vi "_f_SerialComm_Hardware_Module.vi"(5 "Enable(T)":bool=TRUE, 7 "Command":T1, 8 "error in (no error)":errorcluster, 9 "Bytes to read":u32, 10 "Write string":string, 11 "VISA resource name":refnum<visa-resource-name>) -> (0 "error out":errorcluster, 1 "Bytes?":u32, 2 "Read string":string)   [LabVIEW 2013]
uses:
  _f_SerialComm_Hardware_Module Control.ctl
  <vilib>/Instr/_visa.llb/VISA Configure Serial Port (Instr).vi
panel:
  # "Input Data"
  # "Output Data"
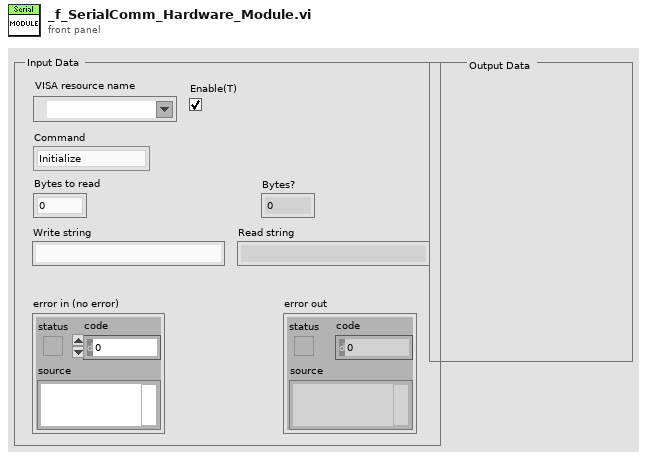
[diagram p1: front panel]
types:
  T1 = typedef "_f_SerialComm_Hardware_Module Control.ctl" = enum16{"Initialize", "Write", "Bytes?", "Read", "Shutdown"}
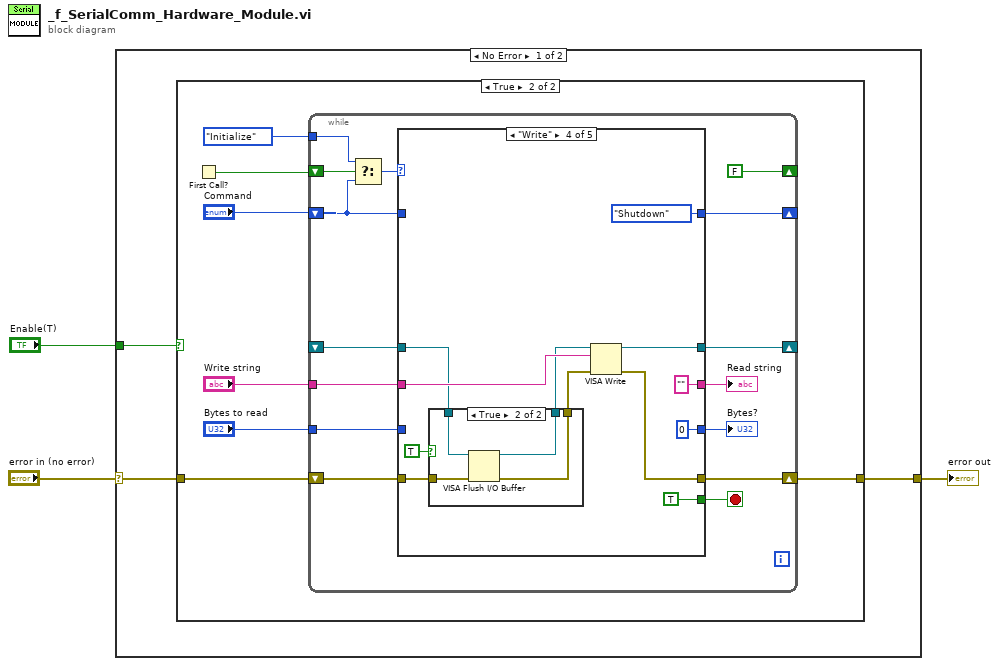
[diagram p0: block diagram]
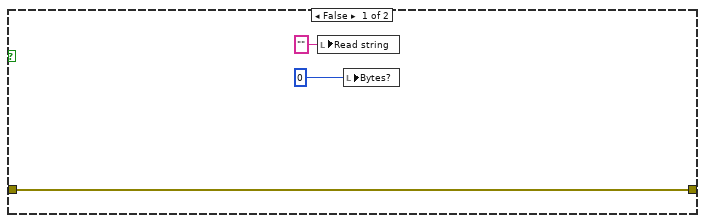
[diagram p2: hidden frame]
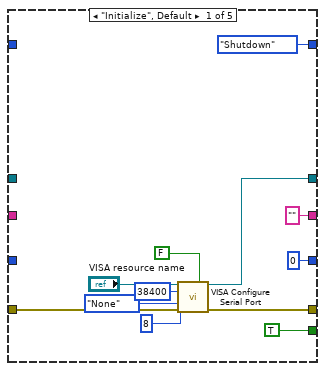
[diagram p3: hidden frame]
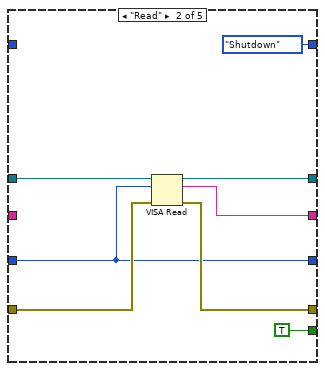
[diagram p4: hidden frame]
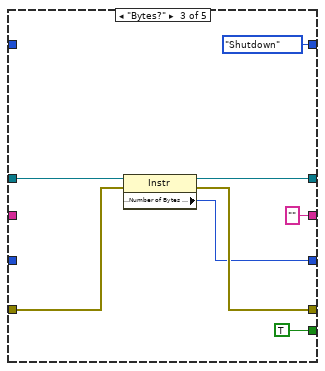
[diagram p5: hidden frame]
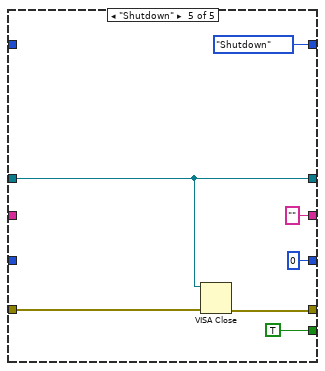
[diagram p7: hidden frame]
diagram:
  n1 = case shown="No Error" "error in (no error)" {
    selector: "error in (no error)" -> [w6 w85]
    tunnel: [w5 w85] -> w2
    tunnel: "Enable(T)" -> [w4 _]
    frame No Error {
      n2 = case shown="True" w4 {
        tunnel: w6 -> [w9 w14]
        tunnel: [w9 w13] -> w5
        frame False {
          n3 = local write "Read string"("" ("Read string")) -> ()
          n4 = local write "Bytes?"(u32 0 ("Bytes?")) -> ()
        }
        frame True {
          n5 = First Call?() -> (First Call?: T/F=w16:bool)
          n6 = while {
            shift-right: [w23] -> _
            shift-left: "Command" -> [w24]
            shift-right: [w26] -> w13
            shift-left: w14 -> [w27]
            shift-right: [FALSE ("First Call?: T/F")] -> _
            shift-left: w16 -> [w31]
            tunnel: _f_SerialComm_Hardware_Module_Control."Initialize" ("t") -> [w30]
            shift-right: [w21] -> _
            shift-left: _ -> [w22]
            tunnel: "Write string" -> [w19]
            tunnel: "Bytes to read" -> [w18]
            stop <- w28 stop-if-true
            n7 = Select(t=w30, s=w31, f=w24) -> (s? t:f=w29:T1)
            n8 = case shown="\"Write\"" w29 {
              tunnel: [TRUE TRUE TRUE TRUE TRUE] -> w28
              tunnel: w27 -> [w34 w45 w54 w65 w84]
              tunnel: [w36 w47 w55 w68 w83] -> w26
              tunnel: w24 -> [_ _ _ _ _]
              tunnel: [_f_SerialComm_Hardware_Module_Control."Shutdown" ("t") _f_SerialComm_Hardware_Module_Control."Shutdown" ("t") _f_SerialComm_Hardware_Module_Control."Shutdown" ("t") _f_SerialComm_Hardware_Module_Control."Shutdown" ("t") _f_SerialComm_Hardware_Module_Control."Shutdown" ("t")] -> w23
              tunnel: w22 -> [_ w46 w57 w66 w82]
              tunnel: [w35 w49 w56 w69 w82] -> w21
              tunnel: ["" ("read buffer") w48 "" ("read buffer") "" ("read buffer") "" ("read buffer")] -> w20
              tunnel: w19 -> [_ _ _ w67 _]
              tunnel: w18 -> [_ w44 _ _ _]
              tunnel: [u32 0 ("Bytes at Port") w44 w53 u32 0 ("Bytes at Port") u32 0 ("Bytes at Port")] -> w17
              frame "Initialize", Default {
                n9 = call-poly "VISA Configure Serial Port"("VISA resource name"="VISA resource name", "Enable Termination\nChar (T)"=FALSE ("Enable Termination\nChar (T)"), "baud rate (9600)"=u32 38400, "data bits (8)"=u16 8, "parity (0:none)"=enum16{"None", "Odd", "Even", "Mark", "Space"}."None", "error in (no error)"=w34) -> ("VISA resource name out"=w35:refnum<visa-resource-name>, "error out"=w36:errorcluster)  [unwired: 8 in]
              }
              frame "Read" {
                n10 = VISA Read(VISA resource name=w46, byte count=w44, error in (no error)=w45) -> (VISA resource name out=w49:refnum<visa-resource-name>, read buffer=w48:string, error out=w47:errorcluster)  [unwired: 1 out]
              }
              frame "Bytes?" {
                n11 = property class="Instr"(reference=w57, error in=w54) -> (reference out=w56:refnum<visa-resource-name>, error out=w55:errorcluster, "Serial Settings:Number of Bytes at Serial Port"=w53:u32)
              }
              frame "Write" {
                n12 = case shown="True" TRUE {
                  tunnel: w66 -> [w72 w77]
                  tunnel: w65 -> [w73 w76]
                  tunnel: [w73 w75] -> w64
                  tunnel: [w72 w74] -> w63
                  frame False {
                  }
                  frame True {
                    n13 = VISA Flush I/O Buffer(VISA resource name=w77, error in (no error)=w76) -> (VISA resource name out=w74:refnum<visa-resource-name>, error out=w75:errorcluster)  [unwired: 1 in]
                  }
                }
                n14 = VISA Write(VISA resource name=w63, write buffer=w67, error in (no error)=w64) -> (VISA resource name out=w69:refnum<visa-resource-name>, error out=w68:errorcluster)  [unwired: 1 out]
              }
              frame "Shutdown" {
                n15 = VISA Close(VISA resource name=w82, error in (no error)=w84) -> (error out=w83:errorcluster)
              }
            }
            "Read string" <- w20
            "Bytes?" <- w17
          }
        }
      }
    }
    frame Error {
    }
  }
  "error out" <- w2
